vi "ApplyModeValues.vi"(0 "reference in":refnum<class "PositionSpeedTest.lvclass">, 5 "error in (no error)":errorcluster) -> (14 "reference out":refnum<class "PositionSpeedTest.lvclass">, 19 "error out":errorcluster)   [LabVIEW 2024, in "PositionSpeedTest.lvclass"]
uses:
  PositionSpeedTest.lvclass
  PositionSpeedTest.lvclass/PositionSpeedTest.ctl
panel:
  # "Connector Pane"
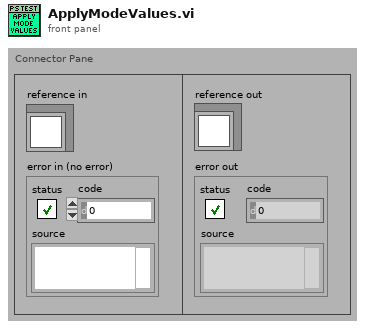
[diagram p1: front panel]
types:
  T1 = enum16{"Test Start", "Test Continue", "Test Failed", "Test Success"}
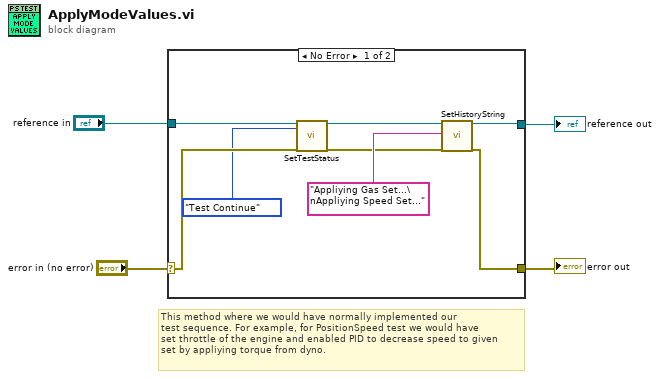
[diagram p0: block diagram]
diagram:
  # "This method where we would have normally implemented our\ntest sequence. For example, for PositionSpeed test we would have\nset throttle of the engine and enabled PID to decrease speed to given\nset by appliying torque from dyno."
  n1 = case shown="No Error" "error in (no error)" {
    selector: "error in (no error)" -> [w12 w14]
    tunnel: [w11 w14] -> w3
    tunnel: [w10 w13] -> w1
    tunnel: "reference in" -> [w7 w13]
    frame No Error {
      n2 = call-dynamic "SetTestStatus.vi"("reference in"=w7, "Test Status"=T1."Test Continue", "error in (no error)"=w12) -> ("reference out"=w6:refnum<class "PositionSpeedTest.lvclass">, "error out"=w8:errorcluster)  [unwired: 15 in]
      n3 = call-dynamic "SetHistoryString.vi"("reference in"=w6, "History String"="Appliying Gas Set...\nAppliying Speed Set..." ("Text"), "error in (no error)"=w8) -> ("reference out"=w10:refnum<class "PositionSpeedTest.lvclass">, "error out"=w11:errorcluster)  [unwired: 15 in]
    }
    frame Error {
    }
  }
  "error out" <- w3
  "reference out" <- w1
